vi "SubVI_TeleOpIntake_TeleOp.vi"(6 "Open/close Intake":bool, 8 "Intake Lift / Lower":bool, 9 "WheelsShootOut":dbl, 10 "WheelsTakeIn":dbl) -> ()   [LabVIEW 2017]
uses:
  <vilib>/Rock Robotics/Network Tables/NT Read Number.vi
panel:
  out "IntakePosition":dbl
  out "Target/actual":cluster{dbl, "Distance":dbl}(graph)
  out "voltage/output":dbl(graph)
  # "e"
  # "1. a\n2. b\n3.x \n4. y\n5. LB \n6. RB\n7. Back\n8 start\n9. LT\n10 RT"
  # "e"
  # "going down"
  # "going up"
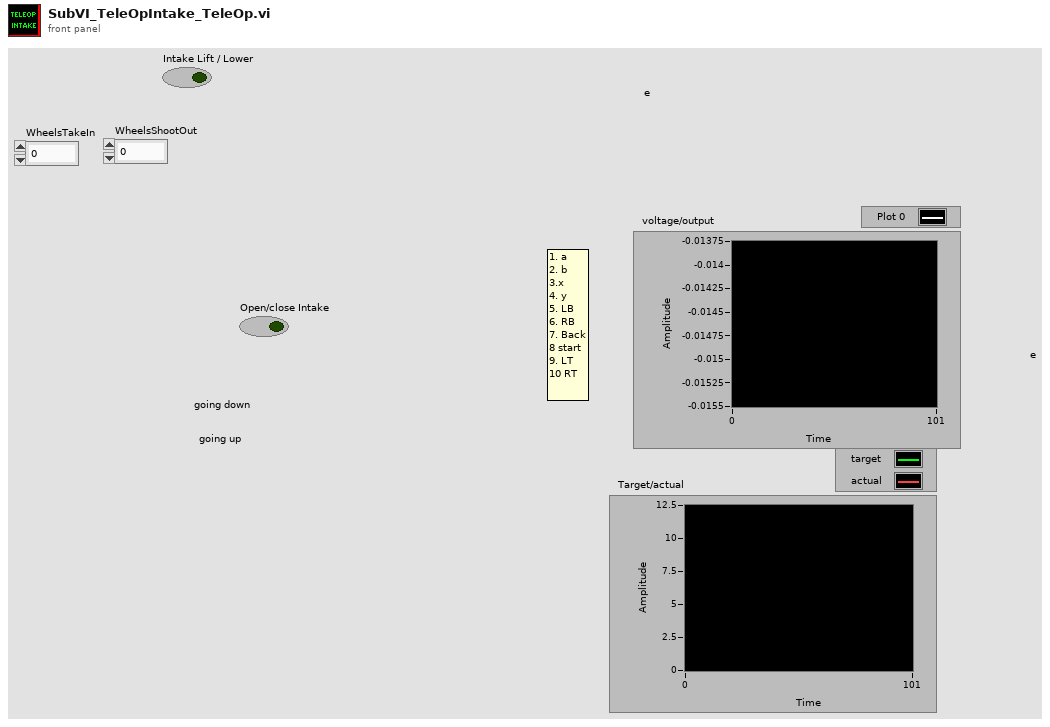
[diagram p1: front panel]
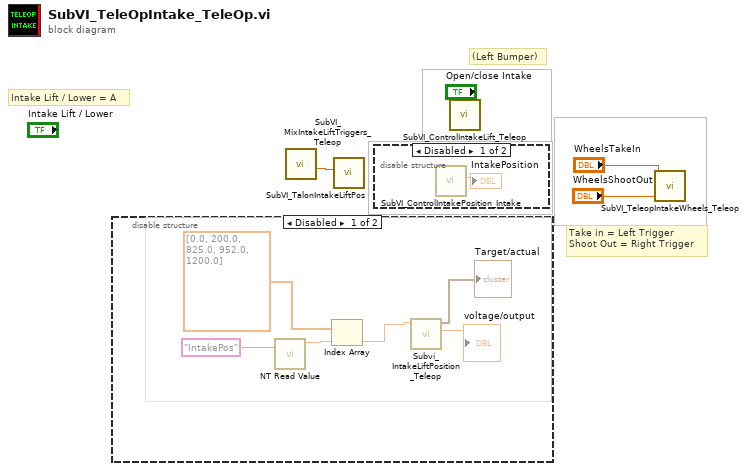
[diagram p0: block diagram]
diagram:
  # "Intake Lift / Lower = A"
  # "Take in = Left Trigger\nShoot Out = Right Trigger"
  # "(Left Bumper)"
  n1 = disable-structure shown="Disabled" {
    frame Disabled {
      n2 = call-poly <vilib>:"NT Read Value.vi"("Name"="IntakePos") -> ("Numeric"=w9:dbl)  [unwired: 9 in, 1 out]
      n3 = Index Array(array=dbl[] [0.0, 200.0, 825.0, 952.0, 1200.0] ("Setpoints"), index=w9) -> (element=w5:dbl)
      n4 = call "Subvi_IntakeLiftPosition_Teleop.vi"("setpoint"=w5) -> ("voltage out"=→"voltage/output":dbl, "Cluster"=→"Target/actual":cluster{"setpoint":dbl, "Distance":dbl})  [unwired: 9 in]
    }
    frame Enabled {
    }
  }
  n5 = call "SubVI_MixIntakeLiftTriggers_Teleop.vi"() -> ("Lift+Lower"=w3:dbl)  [unwired: 11 in]
  n6 = call "SubVI_TalonIntakeLiftPos.vi"("Move Intake position"=w3) -> ()  [unwired: 11 in]
  n7 = disable-structure shown="Disabled" {
    frame Disabled {
      n8 = call "SubVI_ControlIntakePosition_Intake.vi"() -> ("IntakePosition"=→"IntakePosition":dbl, "(IntakeDown)"=w12:bool, "(IntakeUp)"=w13:bool)  [unwired: 9 in]
    }
    frame Enabled {
    }
  }
  n9 = call "SubVI_ControlIntakeLift_Teleop.vi"("Open/close Intake"="Open/close Intake") -> ()  [unwired: 11 in]
  n10 = call "SubVI_TeleopIntakeWheels_Teleop.vi"("WheelsShootOut"="WheelsShootOut", "WheelsTakeIn"="WheelsTakeIn") -> ()  [unwired: 10 in]
